vi "Read RxTx.lvclass.vi"(8 "error in (no error)":errorcluster, 11 "Channel GUI in":refnum<class "Channel GEI.lvclass">) -> (0 "error out":errorcluster, 2 "RxTx.lvclass":refnum<class "RxTx.lvclass">, 3 "Channel GUI out":refnum<class "Channel GEI.lvclass">)   [LabVIEW 2018, in "Channel GEI.lvclass"]
uses:
  Channel GEI.lvclass
  RxTx/RxTx.lvclass
  Channel GEI.lvclass/Channel GEI.ctl
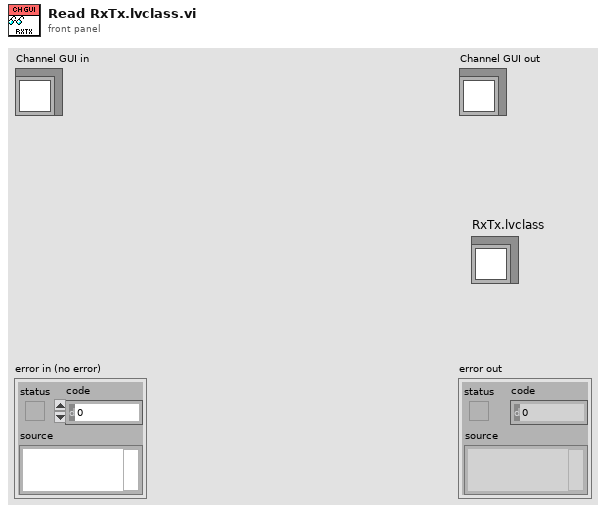
[diagram p1: front panel]
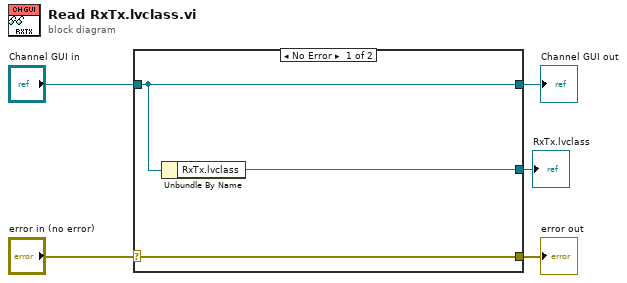
[diagram p0: block diagram]
diagram:
  n1 = case shown="No Error" "error in (no error)" {
    selector: "error in (no error)" -> [w8 w9]
    tunnel: [w8 w9] -> w4
    tunnel: [w6 w10] -> w2
    tunnel: "Channel GUI in" -> [w6 w10]
    tunnel: [w7 _] -> w1
    frame No Error {
      n2 = Unbundle By Name(w6) -> ("RxTx.lvclass"=w7:refnum<class "RxTx.lvclass">)
    }
    frame Error {
    }
  }
  "error out" <- w4
  "Channel GUI out" <- w2
  "RxTx.lvclass" <- w1
